vi "Read_Instr.vi"(8 "error in (no error)":errorcluster caption="entrée d'erreur (pas d'erreur)", 11 "Class Instrument Multimeter en entrée":refnum<class "Class Instrument Balance.lvclass">) -> (0 "error out":errorcluster caption="sortie d'erreur", 3 "Class Instrument Multimeter en sortie":refnum<class "Class Instrument Balance.lvclass">)   [LabVIEW 2020, in "Library Instrument & Equipement.lvlib" / "Library Instruments.lvlib" / "Class Instrument Balance.lvclass"]
uses:
  Class Instrument Balance.lvclass
  Commun VI/TypeDef/Liste Error.ctl
  Class Instrument Balance.lvclass/Class Instrument Balance.ctl
  Instrument (Default)/Class Instrument (Default).lvclass
  Balance/Balance (Default)/Class Balance (Default).lvclass
  Commun VI/Library Commun.lvlib
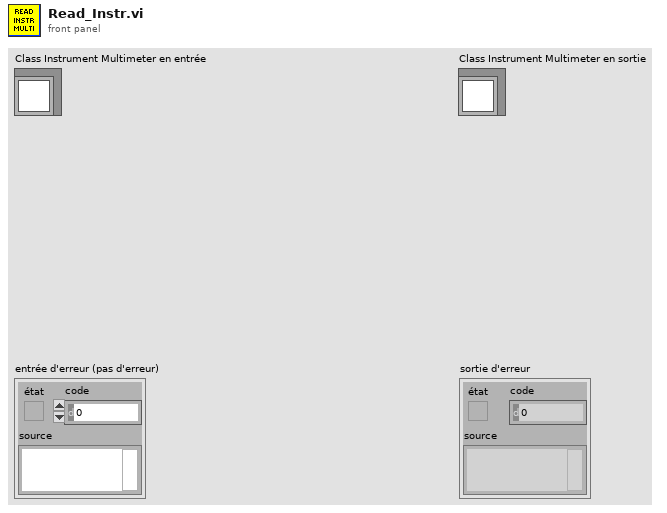
[diagram p1: front panel]
types:
  T1 = typedef "Library Commun.lvlib/Liste Error.ctl" = enum16{"Firebase Driver - Get Document", "Firebase Driver - Get Document With Where", "Firebase Driver - Delete Document", "Firebase Driver - Set Document", "Firebase Driver - Update Document", "Firebase Altyor - Search Document Bench", "Firebase Altyor - Class Not in Firebase", "Spectrum_Analyser - Timeout", "Relay Board - Qty Relay", "DIO - Pb Funtion", "Power_Supply - Peripherical not find", "Mutimeter - Peripherical not find", "Instrument - Function Not Used", "Instrument - Instrument name not specified", "Instrument - Allready Initialised", "Instrument - TimeOut", "Instrument - the instrument must be Initialise before", "Instrument - Frame Not received", "Instrument - Frame Nok", "Test - Initialise the File_for_Save", "Test - Timeout", "Test - Cmd Error", "FGV - Variable ", "BDD FireBase - Define Class", "SN - Class Not Define"}
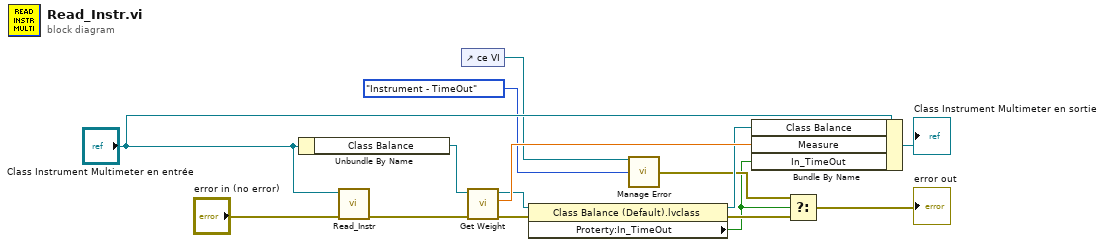
[diagram p0: block diagram]
diagram:
  n1 = Unbundle By Name("Class Instrument Multimeter en entrée") -> ("Class Balance"=w11:refnum<class "Class Balance (Default).lvclass">)
  n2 = call-parent "Read_Instr.vi"("error in (no error)"="error in (no error)", "Class Instrument (Default) en entrée"="Class Instrument Multimeter en entrée") -> ("error out"=w12:errorcluster)  [unwired: 8 in, 1 out]
  n3 = control-ref of="ce VI"() -> (w4:refnum<vi>)
  n4 = call-dynamic "Get Weight.vi"("error in (no error)"=w12, "Class Balance (Default) en entrée"=w11) -> ("error out"=w7:errorcluster, "Get Weight"=w10:dbl, "Class Balance (Default) en sortie"=w9:refnum<class "Class Balance (Default).lvclass">)  [unwired: 7 in]
  n5 = property class="Class Balance (Default).lvclass"(reference=w9, error in=w7) -> (reference out=w8:refnum<class "Class Balance (Default).lvclass">, error out=w5:errorcluster, "Proterty:In_TimeOut"=w1:bool)
  n6 = call "Manage Error.vi"("VI in Error"=w4, "Code Erreur"=Liste_Error."Instrument - TimeOut") -> ("error out"=w2:errorcluster)  [unwired: 13 in]
  n7 = Bundle By Name(cluster="Class Instrument Multimeter en entrée", "Class Balance"=w8, "Measure"=w10, "In_TimeOut"=w1) -> (→"Class Instrument Multimeter en sortie":refnum<class "Class Instrument Balance.lvclass">)
  n8 = Select(t=w2, s=w1, f=w5) -> (s? t:f=→"error out":errorcluster)
